vi "AR7x_Sum.vi"(7 "output":bool, 11 "Cmd In":u8[](array[numeric])) -> (0 "Length":u8 format="%02x", 1 "SUM":u8 format="%02x", 2 "XOR":u8 format="%02x", 3 "Cmd Out":u8[](array[numeric]))   [LabVIEW 2011]
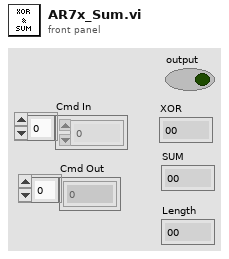
[diagram p1: front panel]
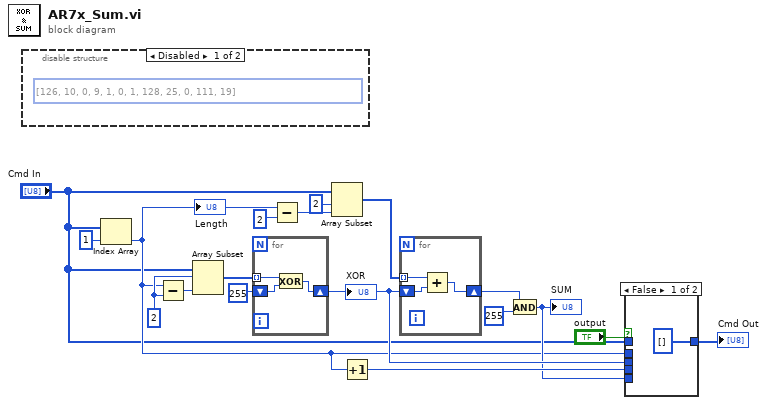
[diagram p0: block diagram]
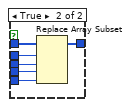
[diagram p2: hidden frame]
diagram:
  w4 = 2 ("index")
  n1 = disable-structure shown="Disabled" {
    frame Disabled {
      (unwired) u8[] [126, 10, 0, 9, 1, 0, 1, 128, 25, 0, 111, 19]
    }
    frame Enabled {
    }
  }
  n2 = Index Array(array="Cmd In", index=1) -> (element=w2:u8)
  "Length" <- w2
  n3 = Subtract(x=w2, y=w4) -> (x-y=w3:i32)
  n4 = Array Subset(array="Cmd In", index=w4, length=w3) -> (w16:u8[])
  n5 = for {
    tunnel: w16 -> [w21] mode=indexing
    shift-right: [w19] -> w8
    shift-left: u8 255 -> [w20]
    n6 = Exclusive Or(1:w20, 2:w21) -> (0:w19:u8)
  }
  "XOR" <- w8
  n7 = Subtract(x=w2, y=u8 2) -> (x-y=w14:u8)
  n8 = Array Subset(array="Cmd In", index=2, length=w14) -> (w12:u8[])
  n9 = Increment(x=w2) -> (x+1=w7:u8)
  n10 = for {
    tunnel: w12 -> [w24] mode=indexing
    shift-right: [w22] -> w11
    shift-left: w8 -> [w23]
    n11 = Add(x=w24, y=w23) -> (x+y=w22:u8)
  }
  n12 = And(x=w11, y=u8 255) -> (x .and. y?=w6:u8)
  "SUM" <- w6
  n13 = case shown="False" "output" {
    tunnel: "Cmd In" -> [_ w31]
    tunnel: w8 -> [_ w30]
    tunnel: w2 -> [_ w29]
    tunnel: w7 -> [_ w28]
    tunnel: w6 -> [_ w27]
    tunnel: [u8[] [] w26] -> w18
    frame False {
    }
    frame True {
      n14 = Replace Array Subset(array=w31, new element #1=w30, index #1=w29, new element #2=w27, index #2=w28) -> (w26:u8[])
    }
  }
  "Cmd Out" <- w18
